vi "SENS_CORR_EXT_AUTO_DCOF.vi"(0 "VISA IN":refnum<visa-resource-name>, 1 "DC Offset ON/OFF":bool, 5 "error in":errorcluster, 7 "Channel":i32) -> (14 "VISA Out":refnum<visa-resource-name>, 19 "error out":errorcluster)   [LabVIEW 2018, in "PNA-X.lvlib"]
doc: "SENSe<cnum>:CORRection:EXTension:AUTO:DCOFfset <bool> \n(Read-Write) Specifies whether or not to include DC Offset as part of automatic port extension. Learn \nmore about Automatic DC Offset. Only allowed when SENS:CORR:EXT:AUTO:LOSS is set to ON. \nParameters \n<cnum> Any existing channel number. If unspecified, value is set to 1 \n<bool> ON (or 1) - Includes DC Offset correction. \nOFF (or 0) - Does NOT include DC Offset correction. \nExamples SENS:CORR:EXT:AUTO:DCOF 1 \nsense2:correction:extension:auto:dcoffset off \nQuery Syntax SENSe<cnum>:CORRection:EXTension:AUTO:DCOFfset? \nReturn Type Boolean \nDefault OFF (0)"
uses:
  PNA-X.lvlib
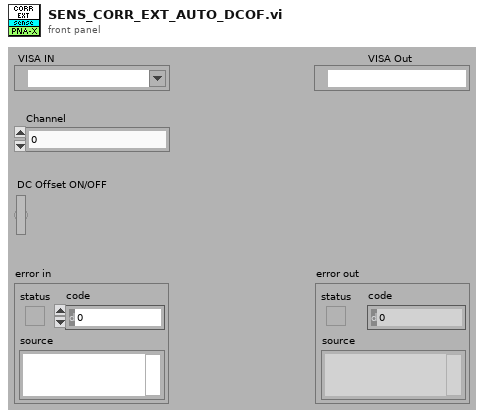
[diagram p1: front panel]
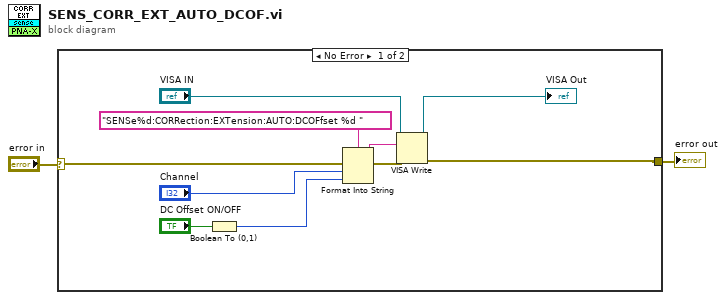
[diagram p0: block diagram]
diagram:
  n1 = case shown="No Error" "error in" {
    selector: "error in" -> [w12 w13]
    tunnel: [w7 w13] -> w1
    frame No Error {
      n2 = Boolean To (0,1)(Boolean="DC Offset ON/OFF") -> (0, 1=w3:i16)
      n3 = Format Into String(format string="SENSe%d:CORRection:EXTension:AUTO:DCOFfset %d " ("Cmdline"), error in=w12, "Channel", w3) -> (resulting string=w10:string, error out=w11:errorcluster)  [unwired: 1 in]
      n4 = VISA Write(VISA resource name="VISA IN", write buffer=w10, error in (no error)=w11) -> (VISA resource name out=→"VISA Out":refnum<visa-resource-name>, error out=w7:errorcluster)  [unwired: 1 out]
    }
    frame Error {
    }
  }
  "error out" <- w1
